vi "Result.Attribute, Convert V2 to Measurement V1 Format.vi"(11 "Attribute":T3 {"Status" items=["LOG", "PASS", "FAIL", "ERROR"]}) -> (3 "Meas":T1 {"Status" items=["LOG", "PASS", "FAIL", "ERROR"]})   [LabVIEW 2018]
uses:
  Result.Attribute.ctl
  Result.Measurement and Attribute Item Status.ctl
  Result.Measurement Item.ctl
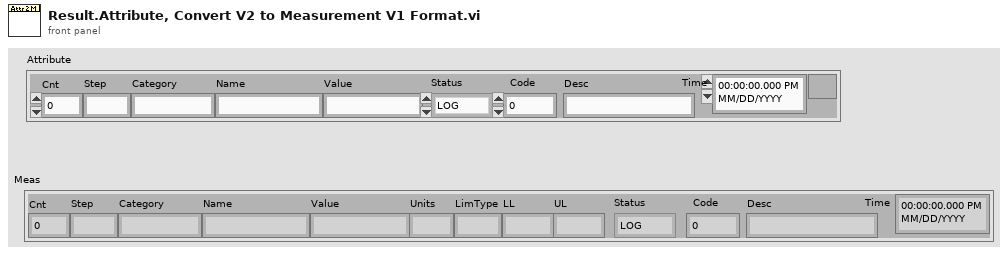
[diagram p1: front panel]
types:
  T1 = typedef "Result.Measurement Item.ctl" = cluster{"Cnt":i32, "Step":string, "Category":string, "Name":string, "Value":string, "Units":string, "LimType":string, "LL":string, "UL":string, "Status":T2, "Code":i32, "Desc":string, "Time":timestamp}
  T2 = typedef "Result.Measurement and Attribute Item Status.ctl" = i32
  T3 = typedef "Result.Attribute.ctl" = cluster{"Cnt":i32, "Step":string, "Category":string, "Name":string, "Value":string, "Status":T2, "Code":i32, "Desc":string, "Time":timestamp}
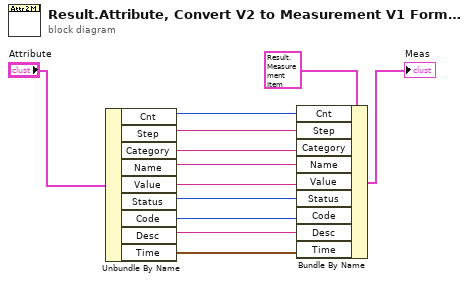
[diagram p0: block diagram]
diagram:
  n1 = Unbundle By Name("Attribute") -> ("Cnt"=w9:i32, "Step"=w8:string, "Category"=w7:string, "Name"=w6:string, "Value"=w5:string, "Status"=w4:T2, "Code"=w3:i32, "Desc"=w2:string, "Time"=w1:timestamp)
  n2 = Bundle By Name(cluster=T1 {"Cnt"=0, "Step"="", "Category"="", "Name"="", "Value"="", "Units"="", "LimType"="", "LL"="", "UL"="", "Status"=0, "Code"=0, "Desc"="", "Time"=timestamp(0 s since 1904-01-01)} ("Meas"), "Cnt"=w9, "Step"=w8, "Category"=w7, "Name"=w6, "Value"=w5, "Status"=w4, "Code"=w3, "Desc"=w2, "Time"=w1) -> (→"Meas":T1)
